vi "CounterSUBVI.vi"() -> ()   [LabVIEW 2015]
panel:
  in  "stop":bool
  out "Numeric":i32
  out "x >= y?":bool
  in  "y":i32=15
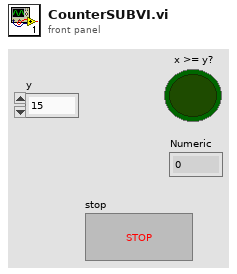
[diagram p1: front panel]
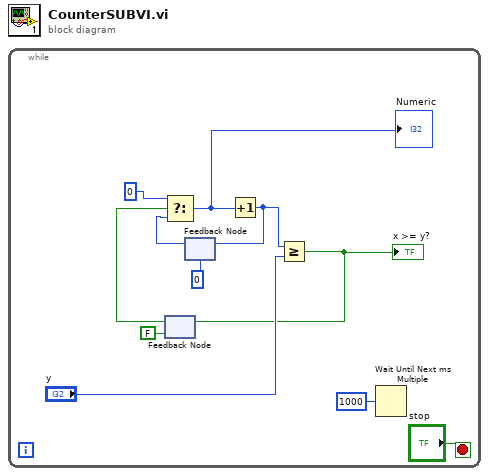
[diagram p0: block diagram]
diagram:
  n1 = while {
    stop <- "stop" stop-if-true
    n2 = feedback #1(FALSE) -> (w8:bool)
    n3 = feedback #2(0) -> (w4:i32)
    n4 = Select(t=0, s=w8, f=w4) -> (s? t:f=w3:i32)
    "Numeric" <- w3
    n5 = Increment(x=w3) -> (x+1=w6:i32)
    n6 = feedback-in #2(w6) -> ()
    n7 = Greater Or Equal?(x=w6, y="y") -> (x >= y?=w9:bool)
    "x >= y?" <- w9
    n8 = feedback-in #1(w9) -> ()
    n9 = Wait Until Next ms Multiple(millisecond multiple=u32 1000) -> ()  [unwired: 1 out]
  }
